vi "JSON to sigs 3.vi"(8 "error in":errorcluster, 11 "JSON string":string) -> (0 "error out":errorcluster, 3 "Signal Sessions":T1)   [LabVIEW 2021]
uses:
  controls/JSON sigs.ctl
  e97f2a44-d1e8-44f2-b915-a6861dd71f71.vi
  <vilib>/JDP Science/JSONtext/JSON text to Variant.vi
  <vilib>/JDP Science/JSONtext/LVClass Serializer/JSONtext LVClass Serializer.lvclass
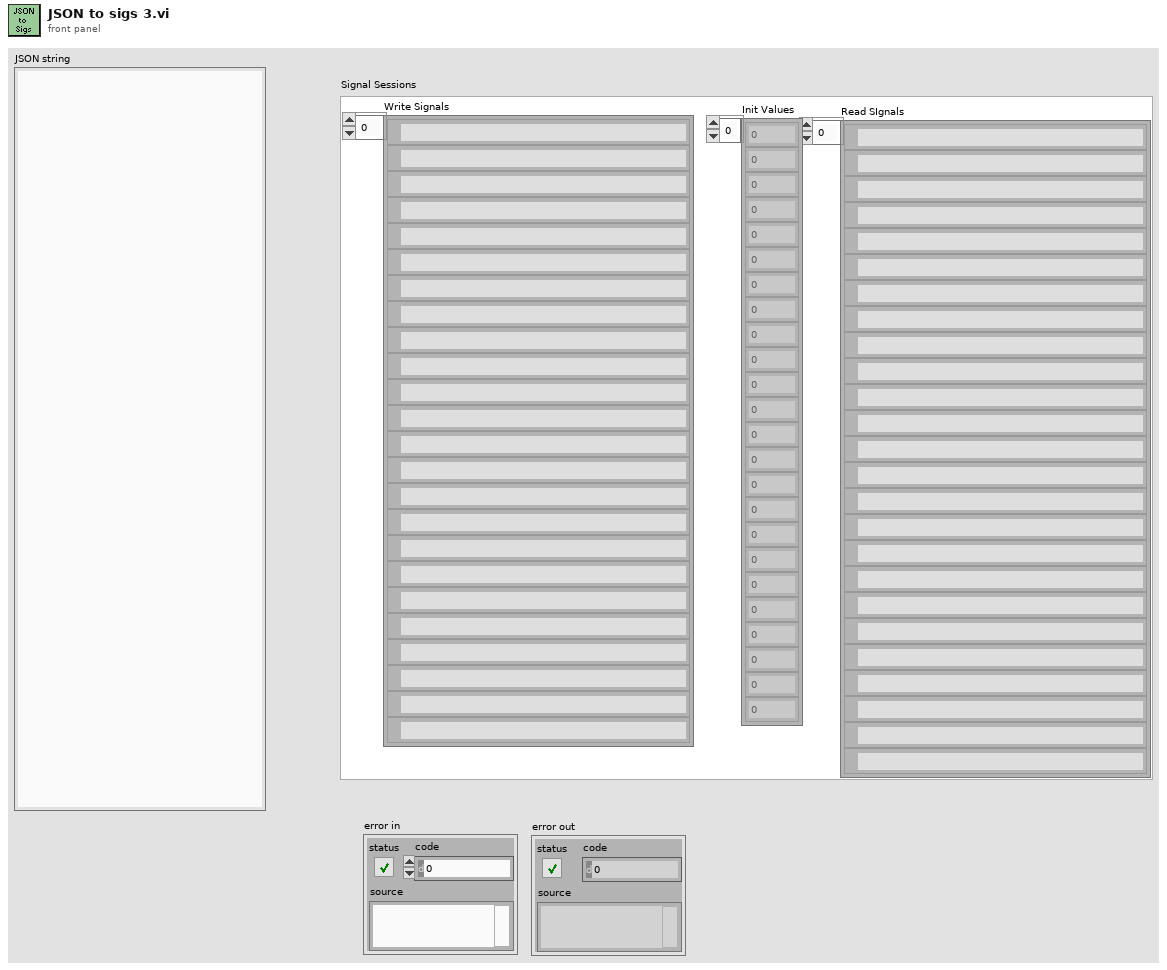
[diagram p1: front panel]
types:
  T1 = typedef "JSON sigs.ctl" = cluster{"Read SIgnals":refnum<k21>[], "Write Signals":refnum<k21>[], "Init Values":dbl[]}
  T2 = cluster{"Write Signals":map{string, i32}, "Read Signals":string}
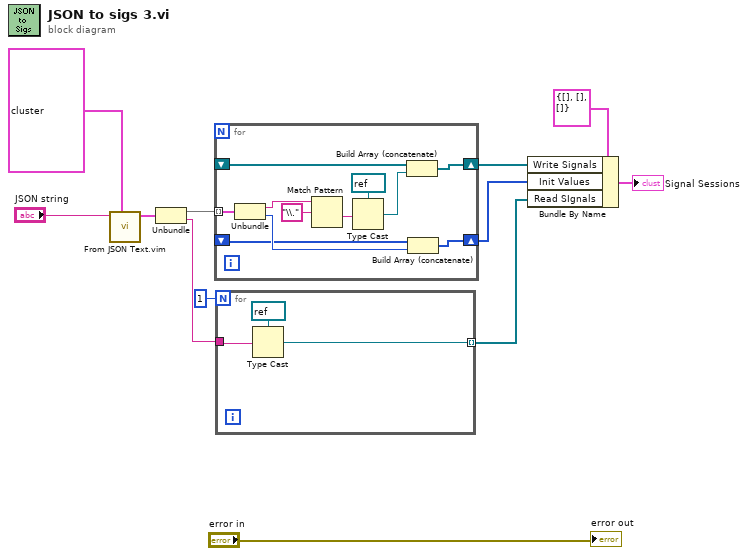
[diagram p0: block diagram]
diagram:
  n1 = call "From JSON Text.vim"("Data Type and Default Value"=T2 {"Write Signals"={}, "Read Signals"=""}, "JSON"="JSON string") -> ("Data out"=w5:T2)  [unwired: 8 in, 1 out]
  n2 = Unbundle(w5) -> ("Write Signals"=w4:map{string, i32}, "Read Signals"=w3:string)
  n3 = for {
    tunnel: w4 -> [w23] mode=indexing
    shift-right: [w17] -> w9
    shift-left: _ -> [w16]
    shift-right: [w18] -> w8
    shift-left: _ -> [w15]
    n4 = Unbundle(w23) -> (w22:string, w19:i32)
    n5 = Match Pattern(string=w22, regular expression="\\.") -> (after substring=w20:string)  [unwired: 1 in, 3 out]
    n6 = Type Cast(type=refnum<k21> refnum ("XNET Signal"), x=w20) -> (*(type *) &x=w14:refnum<k21>)
    n7 = Build Array (concatenate)(w16, w14) -> (w17:refnum<k21>[])
    n8 = Build Array (concatenate)(w15, w19) -> (w18:i32[])
  }
  n9 = for {
    N: 1 -> [_]
    tunnel: w3 -> [w25]
    tunnel: [w24] -> w2 mode=indexing
    n10 = Type Cast(type=refnum<k21> refnum ("XNET Signal"), x=w25) -> (*(type *) &x=w24:refnum<k21>)
  }
  n11 = Bundle By Name(cluster=T1 {"Read SIgnals"=[], "Write Signals"=[], "Init Values"=[]} ("Signal Sessions"), "Write Signals"=w9, "Init Values"=w8, "Read SIgnals"=w2) -> (→"Signal Sessions":T1)
  "error out" <- "error in"
